vi "ManipulateDrive.vi"(4 "Invert":bool, 6 "Y":dbl, 7 "X":dbl) -> (2 "Y":dbl, 3 "X":dbl)   [LabVIEW 2017]
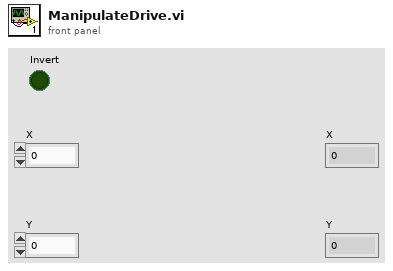
[diagram p1: front panel]
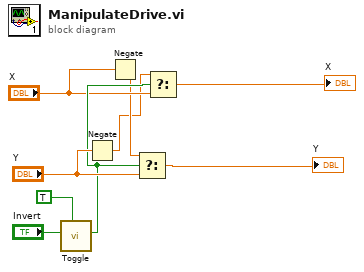
[diagram p0: block diagram]
diagram:
  n1 = call "Toggle.vi"("Control"=TRUE, "Input"="Invert") -> ("Output"=w5:bool)  [unwired: 9 in]
  n2 = Negate(x="Y") -> (-x=w1:dbl)
  n3 = Negate(x="X") -> (-x=w2:dbl)
  n4 = Select(t=w2, s=w5, f="Y") -> (s? t:f=→"Y":dbl)
  n5 = Select(t=w1, s=w5, f="X") -> (s? t:f=→"X":dbl)
